vi "PH_gentec_Powermeter.set Config to GUI.vi"(0 "i ref in":refnum<vi>, 2 "Configuration Values":T1={"Head Type"="", "Head Version"=1, "Serial Number"="", "Calibration Sensitivity"=0.0, "Default Wavelength"=0, "Active Sensitivity"=0.0, "Active Wavelength"=0, "Scale Min Power"=0, "Scale Max Power"=0, "Scale Min Energy"=0, "Scale Max Energy"=0, "Current Scale"=0, "Calo Mode"=FALSE, "Anticipation"=FALSE, "External Trig"=FALSE, "Trig Level"=0.0, "Zero Offset"=0.0, "Multiplier 1"=0.0, "Offset 1"=0.0, "Multiplier 2"=0.0, "Offset 2"=0.0, "Max Power (Joulemeter)"=0.0, "Max energy (Joulemeter)"=0.0, "Currently Logging"=FALSE, "Analog Out Active"=FALSE, "Resolution"=0.0, "Currently Calculating Stats"=FALSE, "High-Resolution Display"=FALSE, "Scale Min Wavelenght"=0, "Scale Max Wavelenght"=0, "Upper Bound"=0.0, "Lower Bond"=0.0, "Reference Value"=0.0, "Thresholds Active"=FALSE, "Fail"=FALSE} {"Reference Value" format="%.6f"; "Lower Bond" format="%.6f"; "Upper Bound" format="%.6f"; "Resolution" format="%.7f"; "Max energy (Joulemeter)" format="%.6f"; "Max Power (Joulemeter)" format="%.6f"; "Offset 2" format="%.6f"; "Multiplier 2" format="%.6f"; "Offset 1" format="%.6f"; "Multiplier 1" format="%.6f"; "Zero Offset" format="%.6f"; "Trig Level" format="%.6f"; "Current Scale" items=["Auto", "1 pJ", "3 pJ", "10 pJ", "30 pJ", "100 pJ", "300 pJ", "1 nJ", "3 nJ", "10 nJ", "30 nJ", "100 nJ", "300 nJ", "1 uJ", "3 uJ", "10 uJ", "30 uJ", "100 uJ", "300 uJ", "1 mJ", "3 mJ", "10 mJ", "30 mJ", "100 mJ", "300 mJ", "1 J", "3 J", "10 J", "30 J", "100 J", "300 J", "1 kJ", "3 kJ", "10 kJ", "30 kJ", "100 kJ", "300 kJ", "1 MJ", "3 MJ", "10 MJ", "30 MJ", "100 MJ", "300 MJ"]; "Scale Max Energy" items=["Auto", "1 pJ", "3 pJ", "10 pJ", "30 pJ", "100 pJ", "300 pJ", "1 nJ", "3 nJ", "10 nJ", "30 nJ", "100 nJ", "300 nJ", "1 uJ", "3 uJ", "10 uJ", "30 uJ", "100 uJ", "300 uJ", "1 mJ", "3 mJ", "10 mJ", "30 mJ", "100 mJ", "300 mJ", "1 J", "3 J", "10 J", "30 J", "100 J", "300 J", "1 kJ", "3 kJ", "10 kJ", "30 kJ", "100 kJ", "300 kJ", "1 MJ", "3 MJ", "10 MJ", "30 MJ", "100 MJ", "300 MJ"]; "Scale Min Energy" items=["Auto", "1 pJ", "3 pJ", "10 pJ", "30 pJ", "100 pJ", "300 pJ", "1 nJ", "3 nJ", "10 nJ", "30 nJ", "100 nJ", "300 nJ", "1 uJ", "3 uJ", "10 uJ", "30 uJ", "100 uJ", "300 uJ", "1 mJ", "3 mJ", "10 mJ", "30 mJ", "100 mJ", "300 mJ", "1 J", "3 J", "10 J", "30 J", "100 J", "300 J", "1 kJ", "3 kJ", "10 kJ", "30 kJ", "100 kJ", "300 kJ", "1 MJ", "3 MJ", "10 MJ", "30 MJ", "100 MJ", "300 MJ"]; "Active Sensitivity" format="%.6f"; "Calibration Sensitivity" format="%.6f"}, 5 "error in":errorcluster) -> (14 "i ref out":refnum<vi>, 19 "error out":errorcluster)   [LabVIEW 2014, in "PH_gentec_Powermeter.lvlib"]
doc: "This VI indicates the wanted Settings at the GUI element."
uses:
  PH_gentec_Powermeter.lvlib
  non_GPL/instr.lib/gentec-SOLO-PE/Driver/Type Defs/gentec-SOLO-PE.Configuration Values.ctl
  non_GPL/instr.lib/gentec-SOLO-PE/Driver/Type Defs/gentec-SOLO-PE.Scale.ctl
  non_GPL/instr.lib/gentec-SOLO-PE/gentec-SOLO-PE - Driver.lvlib
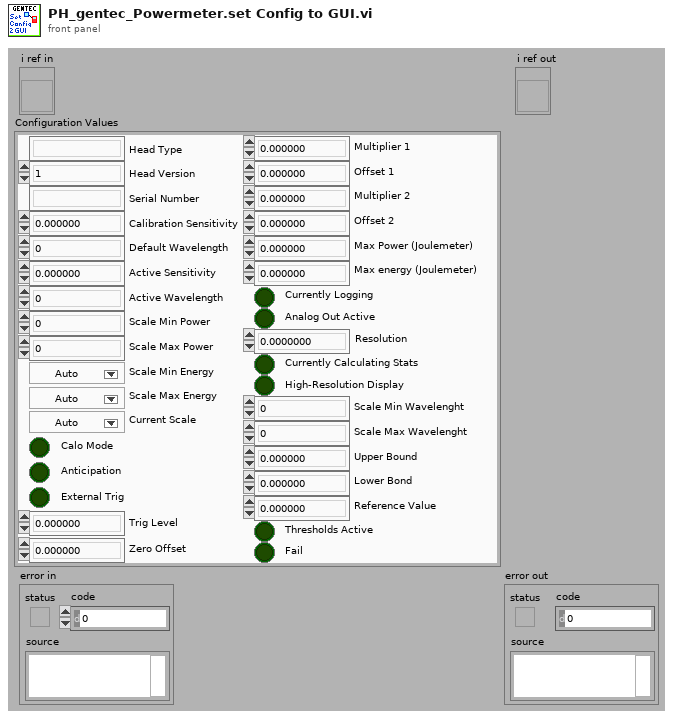
[diagram p1: front panel]
types:
  T1 = typedef "gentec-SOLO-PE - Driver.lvlib/gentec-SOLO-PE.Configuration Values.ctl" = cluster{"Head Type":string, "Head Version":u32, "Serial Number":string, "Calibration Sensitivity":dbl, "Default Wavelength":u32, "Active Sensitivity":dbl, "Active Wavelength":u32, "Scale Min Power":u32, "Scale Max Power":u32, "Scale Min Energy":T2, "Scale Max Energy":T2, "Current Scale":T2, "Calo Mode":bool, "Anticipation":bool, "External Trig":bool, "Trig Level":dbl, "Zero Offset":dbl, "Multiplier 1":dbl, "Offset 1":dbl, "Multiplier 2":dbl, "Offset 2":dbl, "Max Power (Joulemeter)":dbl, "Max energy (Joulemeter)":dbl, "Currently Logging":bool, "Analog Out Active":bool, "Resolution":dbl, "Currently Calculating Stats":bool, "High-Resolution Display":bool, "Scale Min Wavelenght":u32, "Scale Max Wavelenght":u32, "Upper Bound":dbl, "Lower Bond":dbl, "Reference Value":dbl, "Thresholds Active":bool, "Fail":bool}
  T2 = typedef "gentec-SOLO-PE - Driver.lvlib/gentec-SOLO-PE.Scale.ctl" = u32
  T3 = typedef "PH_gentec_Powermeter.lvlib/PH_gentec_Powermeter.i attribute.ctl" = cluster{"GUI References":cluster{"delete":refnum<vi>, "start stop Statistics":refnum<vi>, "Statistic Data":refnum<vi>, "Configuration Values":refnum<vi>, "Set Zero":refnum<vi>, "Data Sampling Settings":refnum<vi>, "Wanted Sets":refnum<vi>, "Current Sets":refnum<vi>}, "Start Stop Statistics":bool, "Wanted Sets":T4, "Current Sets":T4}
  T4 = typedef "PH_gentec_Powermeter.lvlib/PH_gentec_Powermeter.Sets.ctl" = cluster{"Data Sampling Settings":T5, "Set Zero":bool}
  T5 = typedef "gentec-SOLO-PE - Driver.lvlib/gentec-SOLO-PE.Data Sampling Settings.ctl" = cluster{"Sample Rate":u32, "Sample Rate Unit":u32, "Sample Period":u32, "Sample Period Unit":u32, "Total Duration":u32, "Total Duration Unit":u32, "Time Stamp":u32}
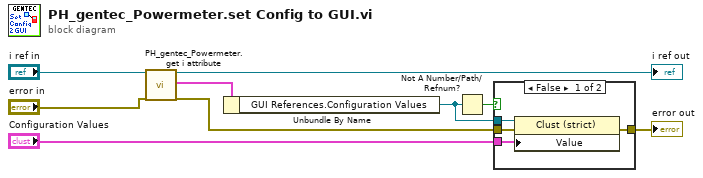
[diagram p0: block diagram]
diagram:
  n1 = call "PH_gentec_Powermeter.get i attribute.vi"("i ref in"="i ref in", "error in (no error)"="error in") -> ("i ref out"=→"i ref out":refnum<vi>, "i attribute"=w8:T3, "error out"=w6:errorcluster)  [unwired: 15 in]
  n2 = Unbundle By Name(w8) -> ("GUI References.Configuration Values"=w4:refnum<vi>)
  n3 = Not A Number/Path/Refnum?(number/path/refnum=w4) -> (NaN/Path/Refnum?=w5:bool)
  n4 = case shown="False" w5 {
    tunnel: [w10 w14] -> w9
    tunnel: w4 -> [w13 _]
    tunnel: w6 -> [w12 w14]
    tunnel: "Configuration Values" -> [w11 _]
    frame False {
      n5 = property class="Clust (strict)"(reference=w13, error in=w12, "Value"=w11) -> (error out=w10:errorcluster)  [unwired: 1 out]
    }
    frame True {
    }
  }
  "error out" <- w9
